vi "Main.vi"() -> ()   [LabVIEW 2019]
uses:
  <vilib>/Platform/TimedLoop/XDataNode/timing_clust.ctl
  <vilib>/Platform/TimedLoop/XDataNode/nitl_modes.ctl
  <vilib>/Platform/TimedLoop/XDataNode/wakeup.ctl
  <vilib>/Analysis/3filter.llb/Filter Passband Type.ctl
  init_var.ctl
  <vilib>/addons/control/pid/pid.llb/PID (DBL).vi
  <vilib>/platform/TimedLoop/XDataNode/XDataNode.xnode
  KNRm_ReMi_OS6_436Motor.lvlibp
  <vilib>/Platform/TimedLoop/XDataNode/XDNodeRunTimeDep.lvlib
  <vilib>/addons/control/pid/NI_PID_pid.lvlib
  <vilib>/ptbypt/NI_PtbyPt.lvlib
  <vilib>/Analysis/NI_AALBase.lvlib
panel:
  in  "步進馬達程式":bool=TRUE
  in  "模擬程式":bool=TRUE
  out "結構是否合理":bool=TRUE
  out "IR":dbl=-23.857993553151026 format="%0.2f"
  out "Stepdeg":dbl=0.19285714285714284 format="%#_2g"
  out "模擬圖":cluster{dbl[], dbl[]}[](graph)=[{[62.44507934888324, 68.04507807993414, 67.49670850165072, 50.0, 62.44507934888324], [50.0, 49.99623008910044, 62.78447824143207, 62.44507934888324, 50.0]}, {array[360 elements], array[360 elements]}, {[33.0, 67.0], [62.11531554372036, 62.774843154046124]}, {[38.25, 38.25], [70.0, 50.0]}]
  in  "Target(+/-)25":dbl(slide)=-25.0 min=25.0 step=1.0 scale=25.0..-25.0 scale format="%#_3g"
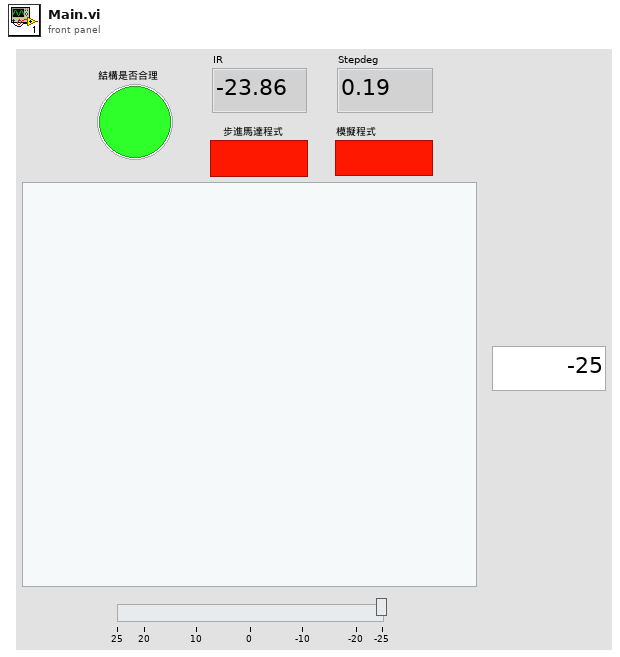
[diagram p1: front panel]
types:
  T1 = typedef "XDNodeRunTimeDep.lvlib/timing_clust.ctl" = cluster{"Expected End [f-1]":u64, "Actual End [f-1]":u64, "Finished Late? [f-1]":bool, "Expected End [i-1]":u64, "Actual End [i-1]":u64, "Finished Late? [i-1]":bool, "Expected Start [i]":u64, "Actual Start [i]":u64, "Expected Start [f]":u64, "Actual Start [f]":u64, "Source Name":string, "Structure Name":string, "Period":i64, "Deadline":i64, "Offset":i64, "Start":i64, "Priority":i32, "Timeout":i32, "Mode":T2, "Wakeup Reason":T3, "Error":errorcluster, "Source Type":string, "Secondary Source Type":string, "Global End Time":u64, "Global Start Time":u64, "Frame Duration":u64, "Iteration Duration":u64, "Assigned CPU":i32, "I/O Scan Engine Mode":u32}
  T2 = typedef "XDNodeRunTimeDep.lvlib/nitl_modes.ctl" = enum32{"No Change", "Process missed periods, maintain original phase", "Discard missed periods, maintain original phase", "Process missed periods, ignore original phase", "Discard missed periods, ignore original phase"}
  T3 = typedef "XDNodeRunTimeDep.lvlib/wakeup.ctl" = enum32{"Normal", "Aborted", "Asynchronous wakeup", "Timing source error", "Timed loop error", "Timeout"}
  T4 = typedef "init_var.ctl" = cluster{"L1":dbl, "L2":dbl, "L3":dbl, "L4":dbl, "θ1":dbl, "θ2":dbl}
  T5 = cluster{"proportional gain (Kc)":dbl, "integral time (Ti, min)":dbl, "derivative time (Td, min)":dbl}
  T6 = typedef "NI_AALBase.lvlib/Filter Passband Type.ctl" = enum32{"Lowpass", "Highpass", "Bandpass", "Bandstop"}
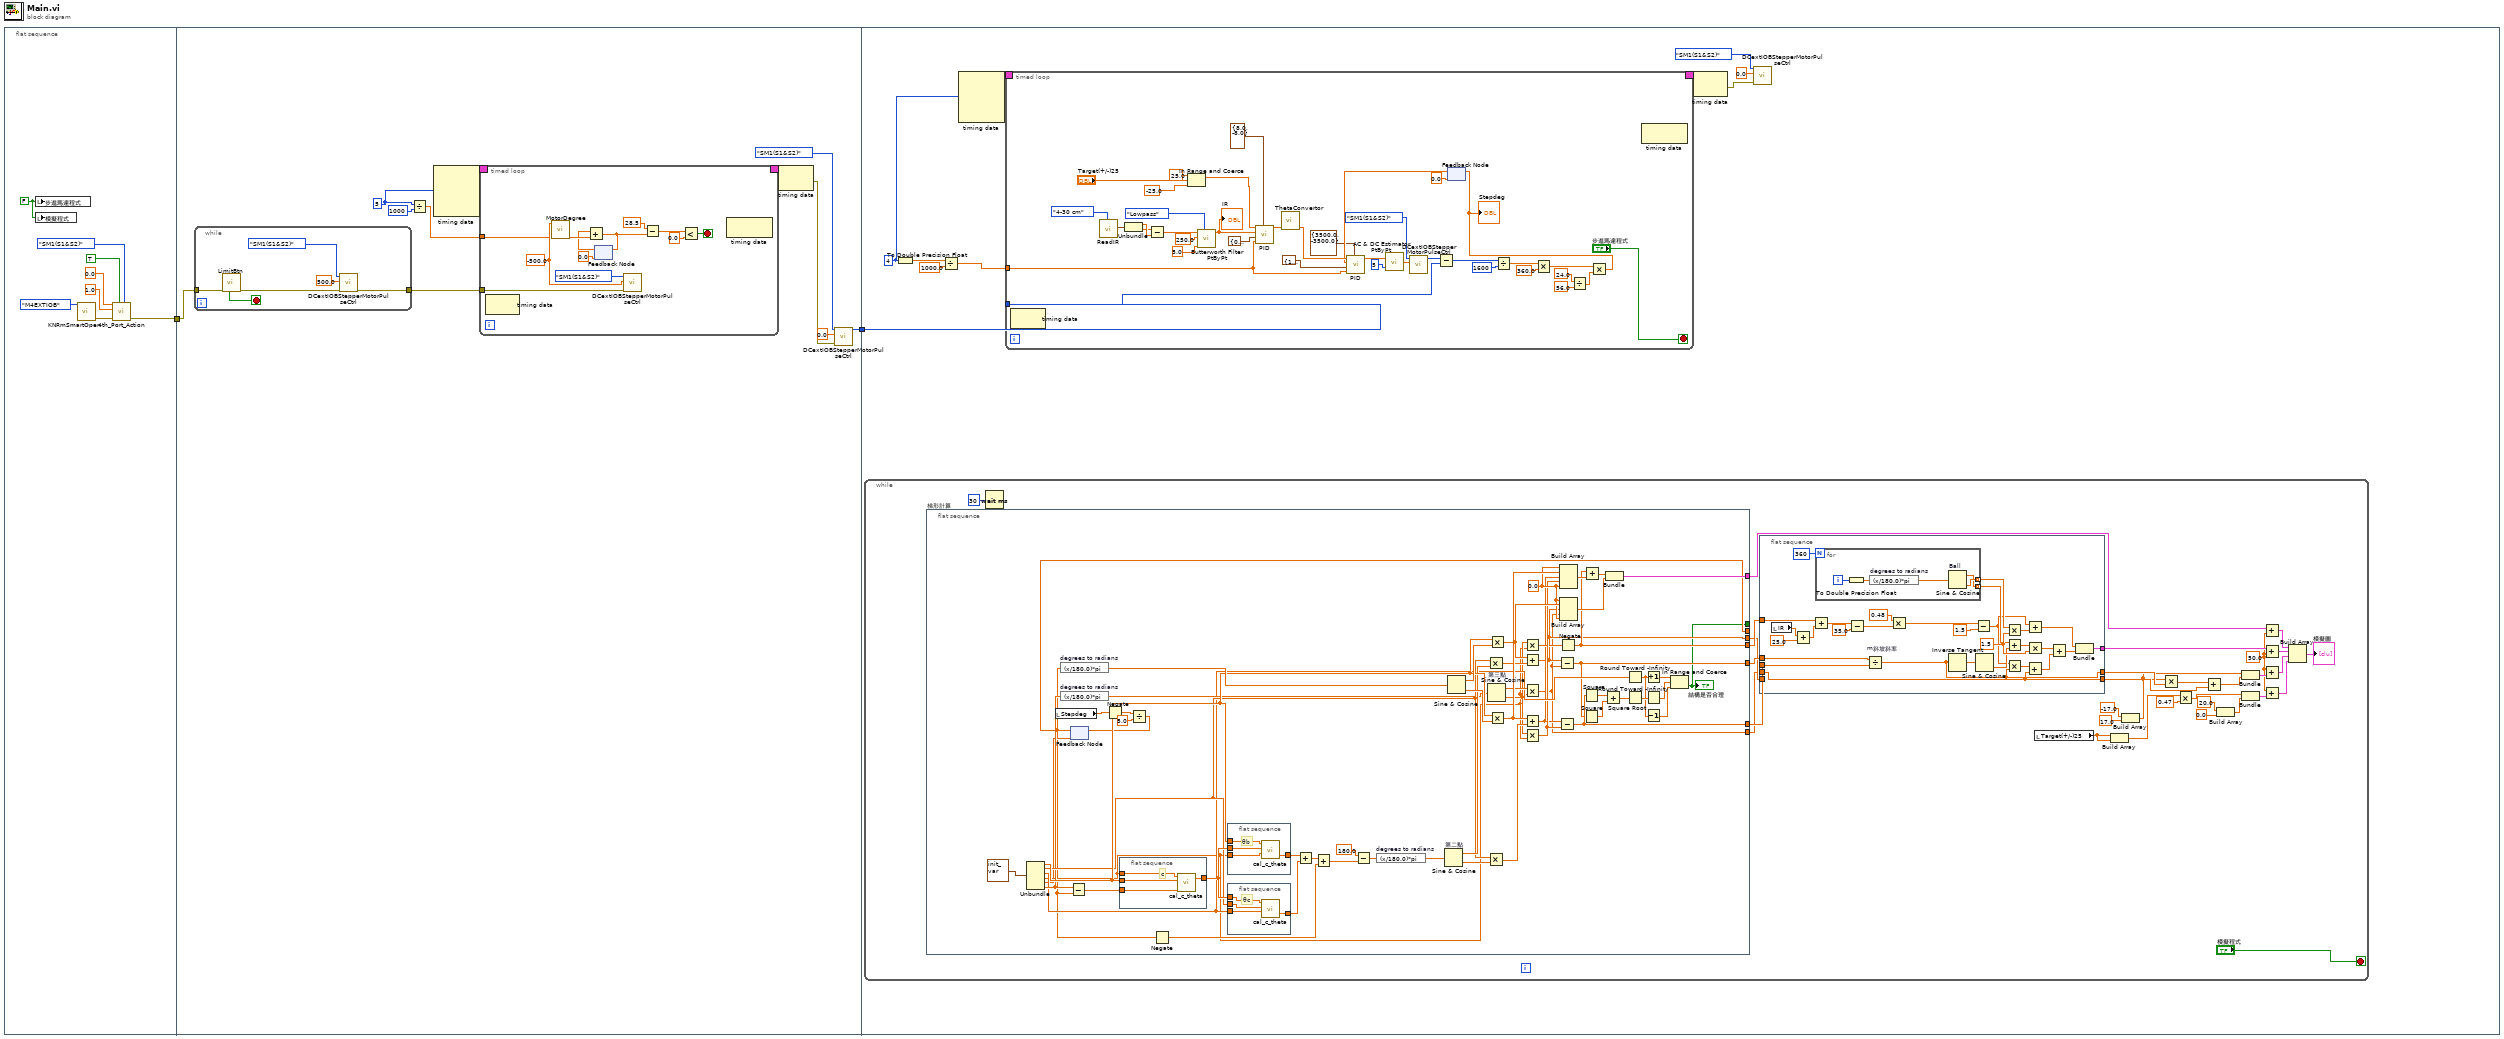
[diagram p0: block diagram]
diagram:
  n1 = flat-sequence {
    tunnel: [w7] -> w1
    tunnel: [w11] -> w2
    tunnel: w1 -> [w20]
    tunnel: w2 -> [w47]
    frame #0 {
      w10 = FALSE ("步進馬達程式")
      n2 = local write "步進馬達程式"(w10) -> ()
      n3 = local write "模擬程式"(w10) -> ()
      n4 = call "KNRmSmartOpen.vi"("INI FPGA MODE"=enum16{"Original", "M4EXTIOB"}."M4EXTIOB") -> ("error out"=w8:errorcluster)  [unwired: 7 in, 3 out]
      n5 = call "4th_Port_Action.vi"("Port"=enum16{"SM1(S1&S2)", "SM2(S3&S4)", "SM3(S5&S6)"}."SM1(S1&S2)", "EN"=TRUE, "error in"=w8, "step"=1.0, "vel(deg/sec)"=0.0) -> ("error out"=w7:errorcluster)  [unwired: 4 in, 2 out]
    }
    frame #1 {
      w17 = i64 5 ("Period")
      n6 = while {
        tunnel: [w45] -> w21
        tunnel: w20 -> [w41]
        stop <- w43 stop-if-true
        n7 = call "LimitBtn.vi"("error in"=w41) -> ("error out"=w42:errorcluster, "LimitBtn"=w43:bool)  [unwired: 9 in]
        n8 = call "DCextIOBStepperMotorPulseCtrl.vi"("error in"=w42, "PulseRate&Dir P/S"=500.0 ("Pulse(Hz) and direction"), "Port"=enum16{"SM1(S1&S2)", "SM2(S3&S4)", "SM3(S5&S6)"}."SM1(S1&S2)") -> ("error out"=w45:errorcluster)  [unwired: 7 in, 1 out]
      }
      n9 = Divide(x=w17, y=i64 1000) -> (x/y=w15:dbl)
      n10 = node-c288(w17) -> (w19:T1)  [unwired: 3 in]
      n11 = timed-loop {
        tunnel: w21 -> [w33]
        timing: w19 -> [_]
        timing-out: [_] -> w18
        tunnel: w15 -> [w26]
        stop <- w29 stop-if-true
        w27 = -500.0 ("Pulse(Hz) and direction")
        n12 = node-c288() -> ()  [unwired: 1 in, 1 out]
        n13 = call "MotorDegree.vi"("Looptime"=w26, "Pulse(Hz) and direction"=w27) -> ("MotorVel"=w25:dbl)  [unwired: 9 in]
        n14 = feedback #1(0.0) -> (w24:dbl)
        n15 = Add(x=w24, y=w25) -> (x+y=w22:dbl)
        n16 = feedback-in #1(w22) -> ()
        n17 = call "DCextIOBStepperMotorPulseCtrl.vi"("error in"=w33, "PulseRate&Dir P/S"=w27, "Port"=enum16{"SM1(S1&S2)", "SM2(S3&S4)", "SM3(S5&S6)"}."SM1(S1&S2)") -> ()  [unwired: 7 in, 2 out]
        n18 = Subtract(x=28.5, y=w22) -> (x-y=w31:dbl)
        n19 = Less?(x=w31, y=0.0) -> (x < y?=w29:bool)
        n20 = node-c288() -> ()  [unwired: 1 in, 1 out]
      }
      n21 = node-c288(w18) -> (w12:errorcluster)
      n22 = call "DCextIOBStepperMotorPulseCtrl.vi"("error in"=w12, "PulseRate&Dir P/S"=0.0, "Port"=enum16{"SM1(S1&S2)", "SM2(S3&S4)", "SM3(S5&S6)"}."SM1(S1&S2)") -> ("PulseCounter+/-"=w11:i32)  [unwired: 7 in, 1 out]
    }
    frame #2 {
      w52 = i64 4 ("Period")
      n23 = while {
        stop <- "模擬程式" stop-if-true
        w61 = 50.0 ("θ1")
        n24 = flat-sequence "梯形計算" {
          tunnel: [w146] -> w82
          tunnel: [w145] -> w86
          tunnel: [w144] -> w85
          tunnel: [w131] -> _
          tunnel: [w125] -> _
          tunnel: [w133] -> w80
          tunnel: [w127] -> w73
          tunnel: [w126] -> w72
          frame #0 {
            w156 = 0.0 ("element")
            n25 = Unbundle(T4 {"L1"=5.6, "L2"=12.8, "L3"=17.5, "L4"=17.6, "θ1"=0.0, "θ2"=135.0} ("初始設定")) -> ("L1"=w167:dbl, "L2"=w164:dbl, "L3"=w147:dbl, "L4"=w136:dbl, "θ1"=w132:dbl, "θ2"=w155:dbl)
            n26 = local read "Stepdeg"() -> (w124:dbl)
            n27 = expression code="(x/180.0)*pi" "degrees to radians"(w155) -> (w154:dbl)
            n28 = feedback #2(w132) -> (w131:dbl)
            n29 = expression code="(x/180.0)*pi" "degrees to radians"(w131) -> (w172:dbl)
            n30 = Subtract(x=w155, y=w131) -> (x-y=w170:dbl)
            n31 = Negate(x=w124) -> (-x=w123:dbl)
            n32 = flat-sequence {
              tunnel: [w189] -> w169
              tunnel: w170 -> [w188]
              tunnel: w136 -> [w187]
              tunnel: w167 -> [w186]
              frame #0 {
                # "c"
                n33 = call "cal_c_theta.vi"("θ"=w188, "b"=w186, "a"=w187) -> ("c"=w189:dbl)  [unwired: 1 in, 1 out]
              }
            }
            n34 = Divide(x=w123, y=5.0 ("x")) -> (x/y=w130:dbl)
            n35 = feedback-in #2(w130) -> ()
            n36 = Negate(x=w131) -> (-x=w152:dbl)
            n37 = flat-sequence {
              tunnel: [w185] -> w177
              tunnel: w167 -> [w184]
              tunnel: w169 -> [w183]
              tunnel: w136 -> [w182]
              frame #0 {
                # "θb"
                n38 = call "cal_c_theta.vi"("c"=w182, "b"=w183, "a"=w184) -> ("theta"=w185:dbl)  [unwired: 1 in, 1 out]
              }
            }
            n39 = flat-sequence {
              tunnel: [w178] -> w176
              tunnel: w169 -> [w181]
              tunnel: w164 -> [w180]
              tunnel: w147 -> [w179]
              frame #0 {
                # "θc"
                n40 = call "cal_c_theta.vi"("c"=w179, "b"=w180, "a"=w181) -> ("theta"=w178:dbl)  [unwired: 1 in, 1 out]
              }
            }
            n41 = Add(x=w177, y=w176) -> (x+y=w173:dbl)
            n42 = Add(x=w173, y=w152) -> (x+y=w174:dbl)
            n43 = Subtract(x=180.0 ("θ1"), y=w174) -> (x-y=w157:dbl)
            n44 = expression code="(x/180.0)*pi" "degrees to radians"(w157) -> (w171:dbl)
            n45 = Sine & Cosine "第二點"(0:w171) -> (1:w165:dbl, 2:w163:dbl)
            n46 = Sine & Cosine(0:w172) -> (1:w168:dbl, 2:w166:dbl)
            n47 = Multiply(x=w164, y=w165) -> (x*y=w159:dbl)
            n48 = Sine & Cosine "第三點"(0:w154) -> (1:w153:dbl, 2:w137:dbl)
            n49 = Multiply(x=w164, y=w163) -> (x*y=w158:dbl)
            n50 = Multiply(x=w167, y=w168) -> (x*y=w160:dbl)
            n51 = Multiply(x=w167, y=w166) -> (x*y=w161:dbl)
            n52 = Multiply(x=w137, y=w136) -> (x*y=w134:dbl)
            n53 = Add(x=w160, y=w159) -> (x+y=w127:dbl)
            n54 = Multiply(x=w153, y=w136) -> (x*y=w126:dbl)
            n55 = Add(x=w161, y=w158) -> (x+y=w128:dbl)
            n56 = Multiply(x=w137, y=w136) -> (x*y=w139:dbl)
            n57 = Subtract(x=w127, y=w126) -> (x-y=w144:dbl)
            n58 = Subtract(x=w128, y=w139) -> (x-y=w145:dbl)
            n59 = Build Array(w156, w161, w128, w139, w156) -> (w138:dbl[])
            n60 = Build Array(w156, w160, w127, w126, w156) -> (w162:dbl[])
            n61 = Negate(x=w134) -> (-x=w133:dbl)
            n62 = Square(x=w145) -> (x^2=w151:dbl)
            n63 = Square(x=w144) -> (x^2=w150:dbl)
            n64 = Add(x=w133, y=w138) -> (x+y=w135:dbl[])
            n65 = Add(x=w151, y=w150) -> (x+y=w149:dbl)
            n66 = Bundle(w135, w162) -> (w146:cluster{dbl[], dbl[]})  [unwired: 1 in]
            n67 = Round Toward -Infinity(1:w147) -> (0:w141:dbl)
            n68 = Square Root(x=w149) -> (sqrt(x)=w148:dbl)
            n69 = Increment(x=w141) -> (x+1=w142:dbl)
            n70 = Round Toward -Infinity(1:w148) -> (0:w143:dbl)
            n71 = Decrement(x=w141) -> (x-1=w140:dbl)
            n72 = In Range and Coerce(upper limit=w142, x=w143, lower limit=w140) -> (In Range?=w125:bool)  [unwired: 1 out]
            "結構是否合理" <- w125
          }
        }
        n73 = Wait (ms)(milliseconds to wait=u32 30) -> ()  [unwired: 1 out]
        n74 = flat-sequence {
          tunnel: w86 -> [w115]
          tunnel: w85 -> [w114]
          tunnel: [w113] -> w84
          tunnel: w80 -> [w101]
          tunnel: [w97] -> w76
          tunnel: w73 -> [_]
          tunnel: w72 -> [w93]
          tunnel: [w93] -> w71
          frame #0 {
            w111 = 1.5 ("θ1")
            n75 = local read "IR"() -> (w90:dbl)
            n76 = Add(x=w90, y=25.0) -> (x+y=w88:dbl)
            n77 = Add(x=w101, y=w88) -> (x+y=w102:dbl)
            n78 = for {
              N: 360 -> [_]
              tunnel: [w118] -> w105 mode=indexing
              tunnel: [w117] -> w110 mode=indexing
              i -> [w120]
              n79 = To Double Precision Float(number=w120) -> (double precision float=w119:dbl)
              n80 = expression code="(x/180.0)*pi" "degrees to radians"(w119) -> (w121:dbl)
              n81 = Sine & Cosine "Ball"(0:w121) -> (1:w117:dbl, 2:w118:dbl)
            }
            n82 = Subtract(x=w102, y=35.0) -> (x-y=w103:dbl)
            n83 = Divide "m斜坡斜率"(x=w114, y=w115) -> (x/y=w97:dbl)
            n84 = Multiply(x=0.48, y=w103) -> (x*y=w98:dbl)
            n85 = Inverse Tangent(1:w97) -> (0:w112:dbl)
            n86 = Subtract(x=w98, y=1.5 ("球位置補償")) -> (x-y=w96:dbl)
            n87 = Sine & Cosine(0:w112) -> (2:w104:dbl)  [unwired: 1 out]
            n88 = Multiply(x=w105, y=w111) -> (x*y=w106:dbl[])
            n89 = Add(x=w110, y=w104) -> (x+y=w108:dbl[])
            n90 = Multiply(x=w96, y=w97) -> (x*y=w95:dbl)
            n91 = Add(x=w95, y=w93) -> (x+y=w94:dbl)
            n92 = Add(x=w96, y=w106) -> (x+y=w99:dbl[])
            n93 = Multiply(x=w108, y=w111) -> (x*y=w109:dbl[])
            n94 = Add(x=w109, y=w94) -> (x+y=w107:dbl[])
            n95 = Bundle(w99, w107) -> (w113:cluster{dbl[], dbl[]})  [unwired: 1 in]
          }
        }
        n96 = local read "Target(+/-)25"() -> (w67:dbl)
        n97 = Build Array(w67, w67) -> (w59:dbl[])
        n98 = Build Array(-17.0 ("element"), 17.0 ("element")) -> (w66:dbl[])
        n99 = Multiply(x=w66, y=w76) -> (x*y=w75:dbl[])
        n100 = Multiply(x=w59, y=0.47 ("element")) -> (x*y=w58:dbl[])
        n101 = Add(x=w75, y=w71) -> (x+y=w74:dbl[])
        n102 = Build Array(20.0 ("element"), 0.0 ("element")) -> (w64:dbl[])
        n103 = Bundle(w66, w74) -> (w79:cluster{dbl[], dbl[]})  [unwired: 1 in]
        n104 = Bundle(w58, w64) -> (w62:cluster{dbl[], dbl[]})  [unwired: 1 in]
        n105 = Add(x=w82, y=w61) -> (x+y=w81:cluster{dbl[], dbl[]})
        n106 = Add(x=w84, y=w61) -> (x+y=w87:cluster{dbl[], dbl[]})
        n107 = Add(x=w61, y=w79) -> (x+y=w69:cluster{dbl[], dbl[]})
        n108 = Add(x=w61, y=w62) -> (x+y=w60:cluster{dbl[], dbl[]})
        n109 = Build Array(w81, w87, w69, w60) -> (→"模擬圖":cluster{dbl[], dbl[]}[])
      }
      n110 = To Double Precision Float(number=w52) -> (double precision float=w54:dbl)
      n111 = Divide(x=w54, y=1000.0) -> (x/y=w51:dbl)
      n112 = node-c288(w52) -> (w56:T1)  [unwired: 3 in]
      n113 = timed-loop {
        timing: w56 -> [_]
        timing-out: [_] -> w55
        tunnel: w51 -> [w208]
        tunnel: w47 -> [w196]
        stop <- "步進馬達程式" stop-if-true
        n114 = node-c288() -> ()  [unwired: 1 in, 1 out]
        n115 = call "ReadIR.vi"("type"=enum16{"10-80 cm", "4-30 cm"}."4-30 cm") -> ("Distance (cm)"=w202:cluster{"IR1":dbl, "IR2":dbl})  [unwired: 8 in, 2 out]
        n116 = Unbundle(w202) -> ("IR1"=w204:dbl, "IR2"=w203:dbl)
        n117 = Subtract(x=w203, y=w204) -> (x-y=w198:dbl)
        n118 = In Range and Coerce(upper limit=25.0, x="Target(+/-)25", lower limit=-25.0) -> (coerced(x)=w192:dbl)  [unwired: 1 out]
        n119 = call <vilib>:"Butterworth Filter PtByPt.vi"("filter type"=Filter_Passband_Type."Lowpass", "low cutoff freq: fl"=5.0, "sampling freq: fs"=250.0, "x"=w198) -> ("Filtered x"=w197:dbl)  [unwired: 5 in, 1 out]
        "IR" <- w197
        n120 = call-poly <vilib>:"PID.vi"("output range"=cluster{"output high":dbl, "output low":dbl} {"output high"=8.0, "output low"=-8.0}, "dt (s)"=w208, "PID gains"=T5 {"proportional gain (Kc)"=0.29999999999999993, "integral time (Ti, min)"=0.03, "derivative time (Td, min)"=0.012999999999999998} ("PosPID"), "process variable"=w197, "setpoint"=w192) -> ("output"=w205:dbl)  [unwired: 5 in, 1 out]
        n121 = call "ThetaConvertor.vi"("Theta2IN"=w205) -> ("Theta1OUT"=w225:dbl)  [unwired: 9 in, 1 out]
        n122 = feedback #3(0.0) -> (w221:dbl)
        n123 = call-poly <vilib>:"PID.vi"("output range"=cluster{"output high":dbl, "output low":dbl} {"output high"=3500.0, "output low"=-3500.0}, "dt (s)"=w208, "PID gains"=T5 {"proportional gain (Kc)"=100.0, "integral time (Ti, min)"=0.0, "derivative time (Td, min)"=0.0} ("StepperPID"), "process variable"=w221, "setpoint"=w225) -> ("output"=w211:dbl)  [unwired: 5 in, 1 out]
        n124 = call <vilib>:"AC & DC Estimator PtByPt.vi"("signal"=w211, "sample length"=5) -> ("DC estimate (V)"=w209:dbl)  [unwired: 1 in, 2 out]
        n125 = call "DCextIOBStepperMotorPulseCtrl.vi"("PulseRate&Dir P/S"=w209, "Port"=enum16{"SM1(S1&S2)", "SM2(S3&S4)", "SM3(S5&S6)"}."SM1(S1&S2)") -> ("PulseCounter+/-"=w213:i32)  [unwired: 8 in, 1 out]
        n126 = Subtract(x=w213, y=w196) -> (x-y=w212:i32)
        n127 = Divide(x=w212, y=1600) -> (x/y=w223:dbl)
        n128 = Multiply(x=w223, y=360.0) -> (x*y=w217:dbl)
        n129 = Divide(x=24.0, y=56.0) -> (x/y=w216:dbl)
        n130 = Multiply(x=w217, y=w216) -> (x*y=w215:dbl)
        "Stepdeg" <- w215
        n131 = feedback-in #3(w215) -> ()
        n132 = node-c288() -> ()  [unwired: 1 in, 1 out]
      }
      n133 = node-c288(w55) -> (w48:errorcluster)
      n134 = call "DCextIOBStepperMotorPulseCtrl.vi"("error in"=w48, "PulseRate&Dir P/S"=0.0 ("Pulse(Hz) and direction"), "Port"=enum16{"SM1(S1&S2)", "SM2(S3&S4)", "SM3(S5&S6)"}."SM1(S1&S2)") -> ()  [unwired: 7 in, 2 out]
    }
  }
